vi "greater than and controlling dial.vi"() -> ()   [LabVIEW 2018]
panel:
  in  "Dial":dbl(knob) scale=0.0..100.0
  out "Numeric 4":dbl
  in  "Numeric 3":dbl
  in  "Numeric 2":dbl
  in  "Numeric":dbl
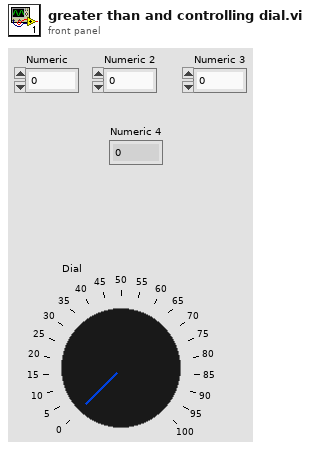
[diagram p1: front panel]
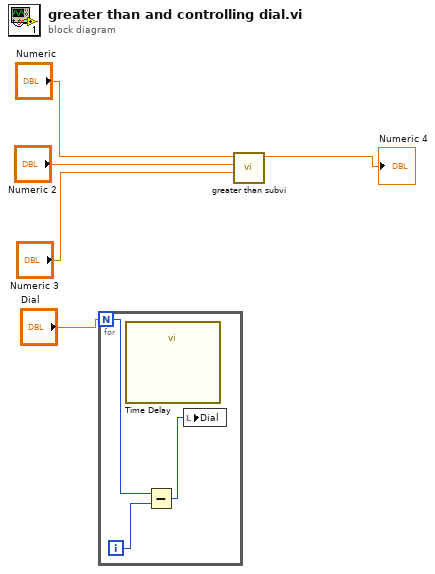
[diagram p0: block diagram]
diagram:
  n1 = for {
    N: "Dial" -> [w7]
    i -> [w8]
    n2 = call "Time Delay"() -> ()  [unwired: 11 in, 1 out]
    n3 = Subtract(x=w7, y=w8) -> (x-y=w6:i32)
    n4 = local write "Dial"(w6) -> ()
  }
  n5 = call "greater than subvi.vi"("Numeric 3"="Numeric 3", "Numeric in"="Numeric 2", "Numeric 4"="Numeric") -> ("Numeric out"=→"Numeric 4":dbl)  [unwired: 8 in]
